vi "Configure LLP Packet Filter.vi"(0 "fpga interface in":refnum<k20>, 5 "data type filter":T1[](array[typedef]), 7 "virtual channel filter":fxp<+,4,4>[](array[numeric]), 11 "error in (no error)":errorcluster, 12 "invert data type filter":bool, 13 "invert virtual channel filter":bool) -> (4 "fpga interface out":refnum<k20>, 15 "error out":errorcluster)   [LabVIEW 2023, in "GettingStarted_Acq_148X_Host.lvlib"]
uses:
  GettingStarted_Acq_148X_Host.lvlib
  <instrlib>/FlexRIO/CSI-2/v2/Common/Types/LLP Data Type.ctl
  Types/148x_Acq_FPGA_Reference.ctl
  <vilib>/Utility/error.llb/Error Cluster From Error Code.vi
  <vilib>/rvi/errors/niLvFpgaAdjustHostInterfaceError.vi
  <vilib>/rvi/interface/nirviReadWriteControl/nirviReadWriteControl.xnode
  <instrlib>/FlexRIO/CSI-2/v2/Host/NI CSI-2 API Host v2.lvlib
  <vilib>/rvi/interface/Simulation/niFpgaSimulationCallBeginRW.vi
  NiFpgaLv.dll
  <instrlib>/FlexRIO/CSI-2/v2/Common/NI CSI-2 API Common v2.lvlib
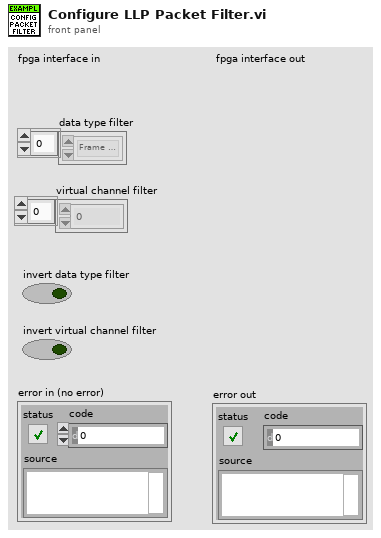
[diagram p1: front panel]
types:
  T1 = typedef "NI CSI-2 API Common v2.lvlib/LLP Data Type.ctl" = enum8{"Frame Start", "Frame End", "Line Start", "Line End", "End of Transmission", "Reserved 0", "Reserved 1", "Reserved 2", "Generic Short Packet 1", "Generic Short Packet 2", "Generic Short Packet 3", "Generic Short Packet 4", "Generic Short Packet 5", "Generic Short Packet 6", "Generic Short Packet 7", "Generic Short Packet 8", "Null", "Blanking Data", "Embedded 8-bit non Image Data", "Generic Long Packet 1", "Generic Long Packet 2", "Generic Long Packet 3", "Generic Long Packet 4", "Reserved 3", "YUV420 8-bit", "YUV420 10-bit", "Legacy YUV420 8-bit", "Reserved 4", "YUV420 8-bit Chroma Shifted", "YUV420 10-bit Chroma Shifted", "YUV422 8-bit", "YUV422 10-bit", "RGB444", "RGB555", "RGB565", "RGB666", "RGB888", "Reserved 5", "Reserved 6", "RAW 24", "RAW 6", "RAW 7", "RAW 8", "RAW 10", "RAW 12", "RAW 14", "RAW 16", "RAW 20", "User Defined 8-bit Data 1", "User Defined 8-bit Data 2", "User Defined 8-bit Data 3", "User Defined 8-bit Data 4", "User Defined 8-bit Data 5", "User Defined 8-bit Data 6", "User Defined 8-bit Data 7", "User Defined 8-bit Data 8", "USL Command", "Reserved 7", "Reserved 8", "Reserved 9", "Reserved 10", "Reserved 11", "Reserved 12", "LRTE EPD Spacer"}
  T2 = typedef "GettingStarted_Acq_148X_Host.lvlib/148x_Acq_FPGA_Reference.ctl" = refnum<k20>
  T3 = cluster{"channel acq config":cluster{"stop timeout (cycles)":u32, "first packet data type select mask":u64, "last packet data type select mask":u64, "first and last packet virtual channel must match":bool}, "virtual channel packet filter mask":u16, "data type packet filter mask":u64, "select corrected csi-2 data":bool, "enable channel":bool}[]
  T4 = cluster{"channel acq config":cluster{"stop timeout (cycles)":u32, "first packet data type select mask":u64, "last packet data type select mask":u64, "first and last packet virtual channel must match":bool}, "virtual channel packet filter mask":u16, "data type packet filter mask":u64, "select corrected csi-2 data":bool, "enable channel":bool}
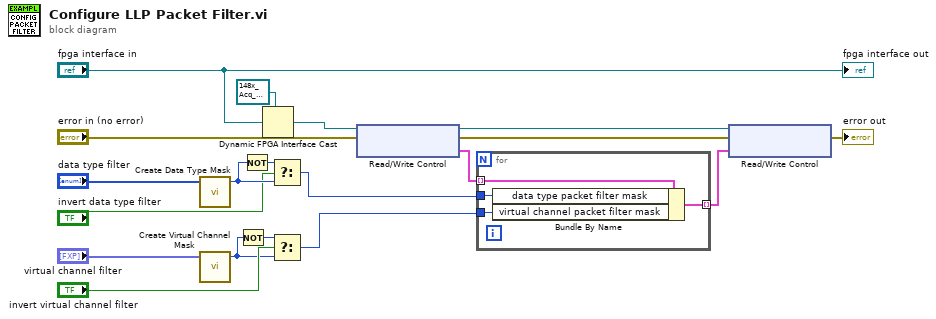
[diagram p0: block diagram]
diagram:
  n1 = call <instrlib>:"Create Data Type Mask.vi"("data types"="data type filter") -> ("data type mask"=w16:u64)  [unwired: 4 in]
  n2 = call <instrlib>:"Create Virtual Channel Mask.vi"("virtual channels"="virtual channel filter") -> ("virtual channel mask"=w18:u16)  [unwired: 4 in]
  n3 = Not(x=w18) -> (.not. x?=w17:u16)
  n4 = Not(x=w16) -> (.not. x?=w14:u64)
  n5 = Dynamic FPGA Interface Cast(Session In=T2 refnum ("FPGA VI Reference Out"), Type="fpga interface in") -> (Session Out=w1:T2)
  n6 = Select(t=w14, s="invert data type filter", f=w16) -> (s? t:f=w3:u64)
  n7 = Select(t=w17, s="invert virtual channel filter", f=w18) -> (s? t:f=w4:u16)
  n8 = xnode "Read/Write Control"("FPGA VI Reference In"=w1, "error in"="error in (no error)") -> ("FPGA VI Reference Out"=w7:T2, "error out"=w8:errorcluster, "channel configs"=w9:T3)
  n9 = for {
    tunnel: w9 -> [w23] mode=indexing
    tunnel: [w22] -> w6 mode=indexing
    tunnel: w4 -> [w21]
    tunnel: w3 -> [w20]
    n10 = Bundle By Name(cluster=w23, "data type packet filter mask"=w20, "virtual channel packet filter mask"=w21) -> (w22:T4)
  }
  n11 = xnode "Read/Write Control"("FPGA VI Reference In"=w7, "error in"=w8, "channel configs"=w6) -> ("error out"=→"error out":errorcluster)  [unwired: 1 out]
  "fpga interface out" <- "fpga interface in"
